vi "Main_v2.vi"() -> ()   [LabVIEW 2019]
doc: "The myRIO Project template acquires acceleration data from the onboard accelerometer and displays the changes of acceleration values in a waveform chart."
uses:
  <vilib>/myRIO/Instrument Drivers/Utilities/Utilities.lvlib
panel:
  out "error out":errorcluster
  in  "Stop":bool
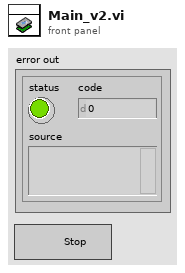
[diagram p1: front panel]
types:
  T1 = enum16{"START", "Inicialización", "Explorar y encontrar tubo", "Desplazarse hacia el tubo", "Acoplar gripper al tubo ", "Dejar marca en tubo", "Desacoplar gripper del tubo", "Girar hasta alinear tubo", "Avanzar sin tocar tubo", "END"}
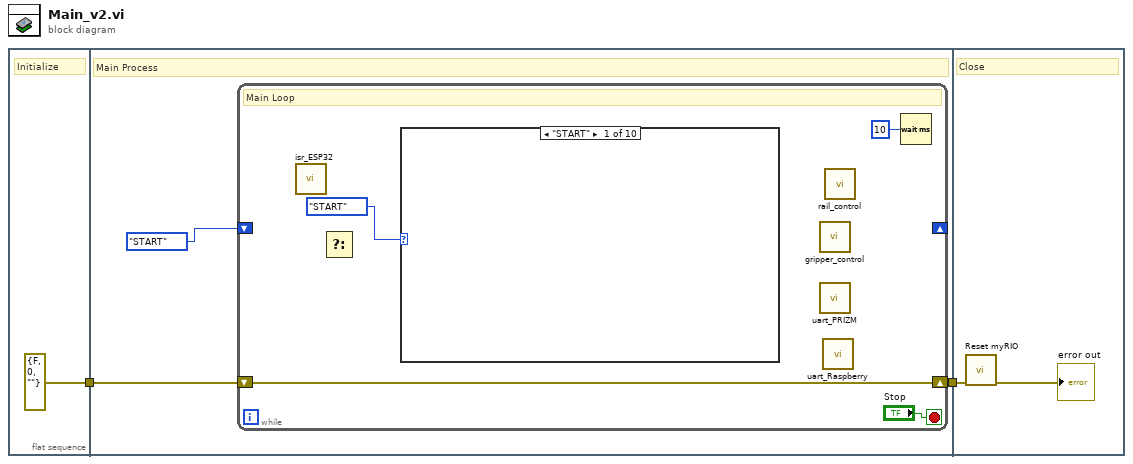
[diagram p0: block diagram]
diagram:
  n1 = flat-sequence {
    tunnel: [errorcluster {"status"=FALSE, "code"=0, "source"=""} ("error in (no error)")] -> w2
    tunnel: w2 -> [w6]
    tunnel: [w5] -> w1
    tunnel: w1 -> [w12]
    frame #0 {
      # "Initialize"
    }
    frame #1 {
      # "Main Process"
      n2 = while {
        shift-right: [w8] -> w5
        shift-left: w6 -> [w8]
        shift-right: _ -> [_]
        shift-left: T1."START" -> [_]
        stop <- "Stop" stop-if-true
        # "Main Loop"
        n3 = call "isr_ESP32.vi"() -> ()  [unwired: 8 in, 1 out]
        n4 = Select() -> ()  [unwired: 3 in, 1 out]
        n5 = case shown="\"START\"" T1."START" {
          frame "START" {
          }
          frame "Inicialización" {
          }
          frame "Explorar y encontrar tubo" {
          }
          frame "Desplazarse hacia el tubo" {
          }
          frame "Acoplar gripper al tubo " {
          }
          frame "Dejar marca en tubo" {
          }
          frame "Desacoplar gripper del tubo" {
          }
          frame "Girar hasta alinear tubo" {
          }
          frame "Avanzar sin tocar tubo" {
          }
          frame "END" {
          }
        }
        n6 = call "gripper_control.vi"() -> ()  [unwired: 3 in, 1 out]
        n7 = call "uart_PRIZM.vi"() -> ()  [unwired: 13 in, 7 out]
        n8 = call "uart_Raspberry.vi"() -> ()  [unwired: 7 in, 5 out]
        n9 = call "rail_control.vi"() -> ()  [unwired: 10 in, 1 out]
        n10 = Wait (ms)(milliseconds to wait=u32 10) -> ()  [unwired: 1 out]
      }
    }
    frame #2 {
      # "Close"
      n11 = call <vilib>:"Reset myRIO.vi"("error in (no error)"=w12) -> ("error out"=→"error out":errorcluster)  [unwired: 10 in]
    }
  }
